vi "Temporary Power.vi"(0 "COM Port in":refnum<visa-resource-name>, 1 "Temporary Power in":dbl=-1.0, 2 "error in":errorcluster) -> (3 "COM Port out":refnum<visa-resource-name>, 4 "OK":bool, 5 "Temporary Power out":dbl, 6 "error out":errorcluster)   [LabVIEW 2013]
doc: "This command sets the laser/led power value.\n\nThe value will NOT be stored in a remanent memory so it will be lost after a reset or after switching mains off. The device will always boot-up with the last value that was set by a “Set Level Power” or “Set Power as Percentage” command.\n\nThis command is intended for use in applications that do need to set new power values continuously (cycles more than 10.000 times per year) to save memory lifetime. The laser/led power value needs to be given as a floating point number from 0.0…100.0.\n\nThe resulting optical power depends on the diode and may be calculated with use of the “Maximum Power” parameter.\n\nTo determine the actual temporary set point value for the optical laser/led power, leave the Temorary Power input unconnected and connect the Temporary Power output instead."
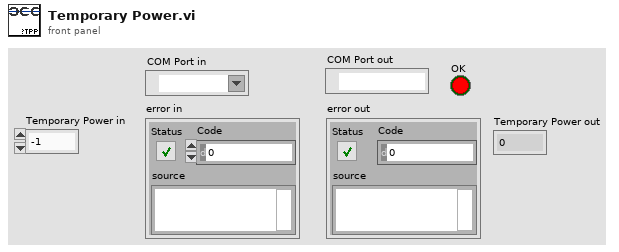
[diagram p1: front panel]
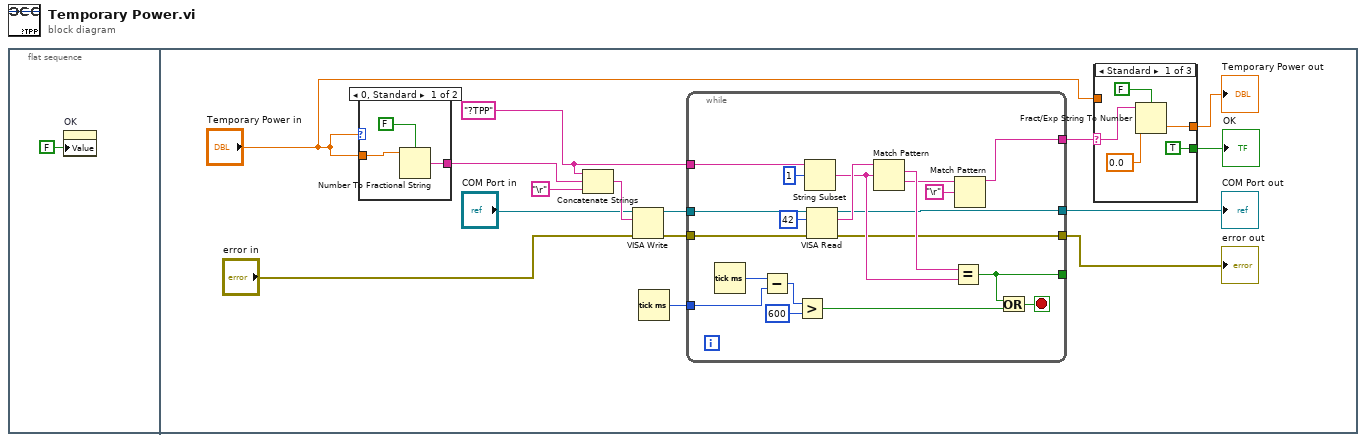
[diagram p0: block diagram]
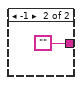
[diagram p2: hidden frame]
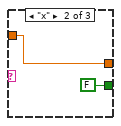
[diagram p3: hidden frame]
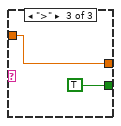
[diagram p4: hidden frame]
diagram:
  n1 = flat-sequence {
    frame #0 {
      n2 = property on="OK" class="Bool. (strikt)"("Value"=FALSE ("OK")) -> ()  [unwired: 2 in, 2 out]
    }
    frame #1 {
      w9 = "?TPP" ("Schreibpuffer")
      n3 = case shown="0, Standard" "Temporary Power in" {
        tunnel: "Temporary Power in" -> [w19 _]
        tunnel: [w18 ""] -> w2
        frame 0, Default {
          n4 = Number To Fractional String(use system decimal point (T)=FALSE ("Systemdezimalzeichen verwenden (T)"), number=w19) -> (F-format string=w18:string)  [unwired: 2 in]
        }
        frame -1 {
        }
      }
      n5 = Concatenate Strings(w9, w2, "\r") -> (w14:string)
      n6 = VISA Write(VISA resource name="COM Port in", write buffer=w14, error in (no error)="error in") -> (VISA resource name out=w11:refnum<visa-resource-name>, error out=w10:errorcluster)  [unwired: 1 out]
      n7 = Tick Count (ms)() -> (millisecond timer value=w8:u32)
      n8 = while {
        tunnel: [w44] -> w16
        tunnel: [w43] -> w15
        tunnel: [w42] -> w7
        tunnel: [w38] -> _
        tunnel: w11 -> [w31]
        tunnel: w10 -> [w40]
        tunnel: w9 -> [w39]
        tunnel: w8 -> [w35]
        stop <- w37 stop-if-true
        n9 = Tick Count (ms)() -> (millisecond timer value=w36:u32)
        n10 = Subtract(x=w36, y=w35) -> (x-y=w34:u32)
        n11 = Greater?(x=w34, y=u32 600) -> (0:w32:bool)
        n12 = String Subset(string=w39, offset (0)=1 ("Offset (0)")) -> (substring=w45:string)  [unwired: 1 in]
        n13 = VISA Read(VISA resource name=w31, byte count=u32 42 ("Byte-Anzahl"), error in (no error)=w40) -> (VISA resource name out=w44:refnum<visa-resource-name>, read buffer=w48:string, error out=w43:errorcluster)  [unwired: 1 out]
        n14 = Match Pattern(string=w48, regular expression=w45) -> (match substring=w47:string, after substring=w41:string)  [unwired: 1 in, 2 out]
        n15 = Equal?(x=w47, y=w45) -> (x = y?=w38:bool)
        n16 = Match Pattern(string=w41, regular expression="\r") -> (before substring=w42:string)  [unwired: 1 in, 3 out]
        n17 = Or(x=w38, y=w32) -> (x .or. y?=w37:bool)
      }
      "COM Port out" <- w16
      "error out" <- w15
      n18 = case shown="Standard" w7 {
        selector: w7 -> [w24 _ _]
        tunnel: [TRUE FALSE TRUE] -> w6
        tunnel: [w23 w26 w28] -> w4
        tunnel: "Temporary Power in" -> [_ w26 w28]
        frame Default {
          n19 = Fract/Exp String To Number(use system decimal point (T)=FALSE ("Systemdezimalzeichen verwenden (T)"), string=w24, default (0 dbl)=0.0 ("Standard (0 I32)")) -> (number=w23:dbl)  [unwired: 1 in, 1 out]
        }
        frame "x" {
        }
        frame ">" {
        }
      }
      "OK" <- w6
      "Temporary Power out" <- w4
    }
  }
